vi "Calculate Required Steering Angle.vi"(7 "constraint error tolerance (1E-12)":dbl=1e-12, 8 "error in (no error)":errorcluster, 9 "wheel frame velocity":dbl[](array[numeric]), 11 "steering wheel in":refnum<class "NI_Robotics_Steering Wheel.lvclass">) -> (0 "error out":errorcluster, 2 "required steering angle (rad)":dbl, 3 "steering wheel out":refnum<class "NI_Robotics_Steering Wheel.lvclass">)   [LabVIEW 2017, in "NI_Robotics_Steering Wheel.lvclass"]
uses:
  <vilib>/robotics/Steering/Steering Wheel/NI_Robotics_Steering Wheel.lvclass
  c:/Program Files (x86)/National Instruments/LabVIEW 2017/vi.lib/robotics/Steering/Wheel/NI_Robotics_Wheel.lvclass
  <vilib>/robotics/Steering/Steering Wheel/NI_Robotics_Steering Wheel.lvclass/NI_Robotics_Steering Wheel.ctl
  <vilib>/robotics/Steering/Wheel/NI_Robotics_Wheel.lvclass/NI_Robotics_Wheel.ctl
  <vilib>/Analysis/coordinate.llb/Angle Rotation (scalar).vi
  <vilib>/Analysis/coordinate.llb/Check for Included Angle (scalar).vi
  <vilib>/Analysis/coordinate.llb/Absolute Angle Difference (scalar).vi
  <vilib>/Analysis/coordinate.llb/Wrap Angle (scalar).vi
  <vilib>/Analysis/coordinate.llb/Set Angle Unit.vi
  <vilib>/robotics/Steering/Wheel/NI_Robotics_Wheel.lvclass
  <vilib>/robotics/Utilities/NI_Robotics Utilities.lvlib
  <vilib>/Analysis/NI_AAL_Angle.lvlib
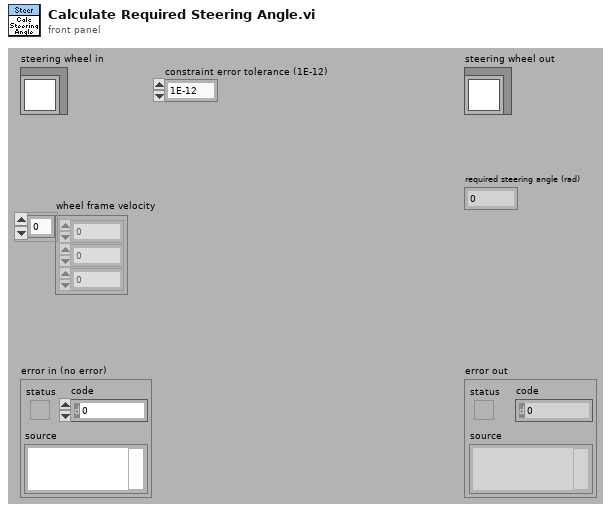
[diagram p1: front panel]
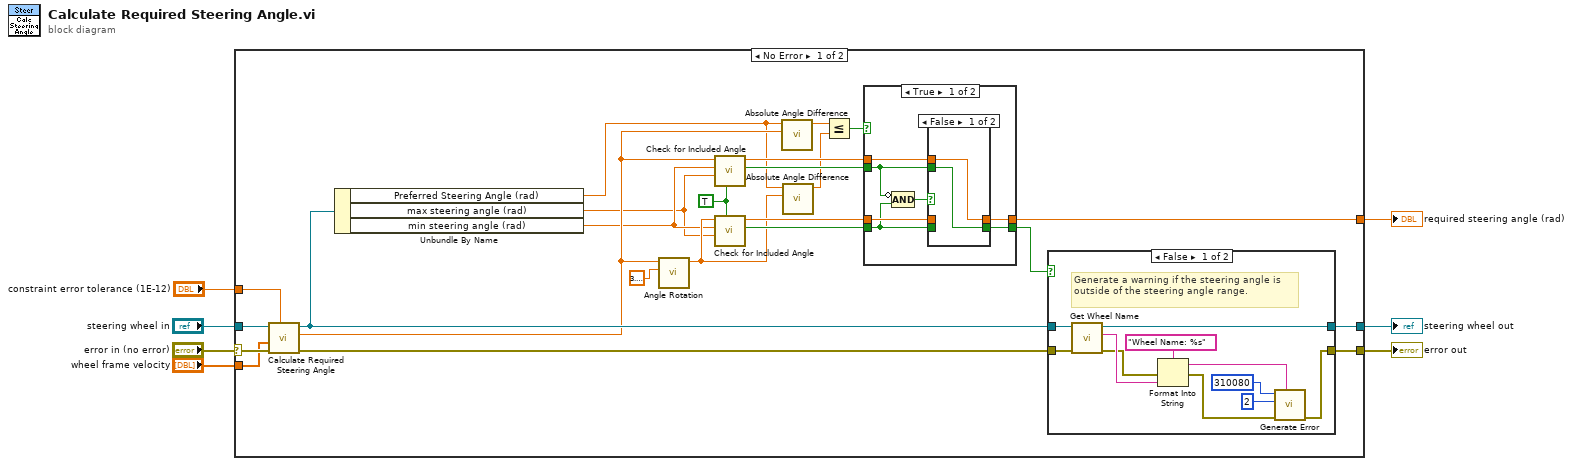
[diagram p0: block diagram]
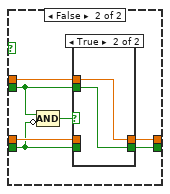
[diagram p3: hidden frame]
diagram:
  n1 = case shown="No Error" "error in (no error)" {
    selector: "error in (no error)" -> [w31 w68]
    tunnel: "wheel frame velocity" -> [w29 _]
    tunnel: "steering wheel in" -> [w30 w67]
    tunnel: "constraint error tolerance (1E-12)" -> [w28 _]
    tunnel: [w26 w68] -> w3
    tunnel: [w24 w67] -> w2
    tunnel: [w21 _] -> w1
    frame No Error {
      w15 = TRUE ("coerce output (F)")
      n2 = call-parent "Calculate Required Steering Angle.vi"("constraint error tolerance (1E-12)"=w28, "error in (no error)"=w31, "wheel frame velocity"=w29, "wheel in"=w30) -> ("error out"=w27:errorcluster, "required steering angle (rad)"=w14:dbl, "wheel out"=w25:refnum<class "NI_Robotics_Steering Wheel.lvclass">)  [unwired: 5 in]
      n3 = Unbundle By Name(w25) -> ("Preferred Steering Angle (rad)"=w12:dbl, "max steering angle (rad)"=w8:dbl, "min steering angle (rad)"=w9:dbl)
      n4 = call-poly <vilib>:"Angle Rotation.vi"("counterclockwise rotation"=3.141592653589793, "angle"=w14) -> ("rotated angle"=w11:dbl)  [unwired: 8 in, 1 out]
      n5 = call-poly <vilib>:"Check for Included Angle.vi"("coerce angle"=w15, "end angle"=w8, "start angle"=w9, "angle in"=w14) -> ("in range?"=w16:bool, "angle out"=w17:dbl)  [unwired: 5 in, 1 out]
      n6 = call-poly <vilib>:"Check for Included Angle.vi"("coerce angle"=w15, "end angle"=w8, "start angle"=w9, "angle in"=w11) -> ("in range?"=w18:bool, "angle out"=w19:dbl)  [unwired: 5 in, 1 out]
      n7 = call-poly <vilib>:"Absolute Angle Difference.vi"("angle 2"=w14, "angle 1"=w12) -> ("absolute angle difference"=w13:dbl)  [unwired: 8 in, 1 out]
      n8 = call-poly <vilib>:"Absolute Angle Difference.vi"("angle 2"=w11, "angle 1"=w12) -> ("absolute angle difference"=w10:dbl)  [unwired: 8 in, 1 out]
      n9 = Less Or Equal?(x=w13, y=w10) -> (x <= y?=w23:bool)
      n10 = case shown="True" w23 {
        tunnel: w16 -> [w36 w47]
        tunnel: w17 -> [w37 w48]
        tunnel: w19 -> [w35 w46]
        tunnel: w18 -> [w34 w45]
        tunnel: [w33 w44] -> w21
        tunnel: [w32 w43] -> w22
        frame True {
          n11 = Compound Arithmetic op=AND(invert w36, w34) -> (w38:bool)
          n12 = case shown="False" w38 {
            tunnel: w37 -> [w40 _]
            tunnel: w36 -> [w39 _]
            tunnel: w35 -> [_ w42]
            tunnel: w34 -> [_ w41]
            tunnel: [w40 w42] -> w33
            tunnel: [w39 w41] -> w32
            frame False {
            }
            frame True {
            }
          }
        }
        frame False {
          n13 = Compound Arithmetic op=AND(w47, invert w45) -> (w49:bool)
          n14 = case shown="True" w49 {
            tunnel: w48 -> [_ w53]
            tunnel: w47 -> [_ w52]
            tunnel: w46 -> [w51 _]
            tunnel: w45 -> [w50 _]
            tunnel: [w51 w53] -> w44
            tunnel: [w50 w52] -> w43
            frame False {
            }
            frame True {
            }
          }
        }
      }
      n15 = case shown="False" w22 {
        tunnel: w27 -> [w56 w66]
        tunnel: [w62 w66] -> w26
        tunnel: w25 -> [w58 w65]
        tunnel: [w55 w65] -> w24
        frame False {
          # "Generate a warning if the steering angle is outside of the steering angle range."
          n16 = call <vilib>:"Get Wheel Name.vi"("error in (no error)"=w56, "wheel in"=w58) -> ("error out"=w59:errorcluster, "wheel name"=w60:string, "wheel out"=w55:refnum<class "NI_Robotics_Steering Wheel.lvclass">)  [unwired: 7 in]
          n17 = Format Into String(format string="Wheel Name: %s", error in=w59, w60) -> (resulting string=w54:string, error out=w57:errorcluster)  [unwired: 1 in]
          n18 = call <vilib>:"Generate Error.vi"("<append> (\"\")"=w54, "error in (no error)"=w57, "chain levels to remove (1)"=2, "code"=310080) -> ("error out"=w62:errorcluster)  [unwired: 7 in]
        }
        frame True {
        }
      }
    }
    frame Error {
    }
  }
  "error out" <- w3
  "steering wheel out" <- w2
  "required steering angle (rad)" <- w1
